vi "SANM_FreqMod.vi"() -> ()   [LabVIEW 2012]
panel:
  out "f":fxp<+/-,32,0>
  in  "K":fxp<+,16,0>
  in  "Nominal Freq":fxp<+,16,0>
  in  "Decimation":i16
  in  "Stages":i16
  in  "Dec1":i16
  in  "Dec2":i16
  out "ChannelQ":i64
  out "ChannelI":i64
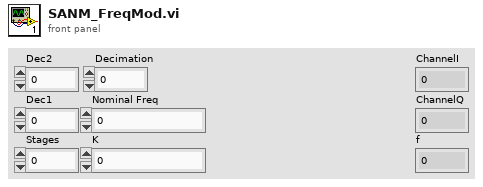
[diagram p1: front panel]
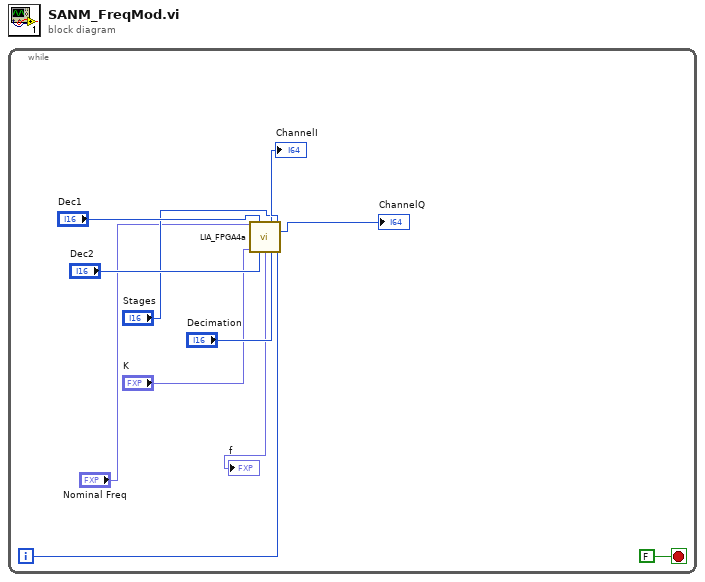
[diagram p0: block diagram]
diagram:
  n1 = while {
    i -> [w1]
    stop <- FALSE stop-if-true
    n2 = call "LIA_FPGA4a.vi"("nominal freq"="Nominal Freq", "dec1"="Dec1", "stages"="Stages", "K"="K", "dec2"="Dec2", "decimation"="Decimation", "While Loop Counter"=w1) -> ("channelI"=→"ChannelI":i64, "channelQ"=→"ChannelQ":i64, "f"=→"f":fxp<+/-,32,0>)  [unwired: 4 in, 2 out]
  }
